vi "Configure Dialog.vi"(2 "First time?":bool) -> ()   [LabVIEW 2016]
uses:
  Communication Global variables.vi
panel:
  in  "REST URL":string="http://10.27.67.2:5800"
  in  "Cancel Button":bool
  in  "Save":bool
  in  "UDP Port":u16=5803
  in  "Robot IP Address":string="10.27.67.2"
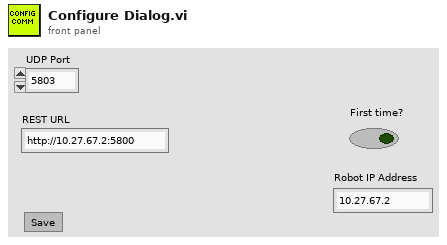
[diagram p1: front panel]
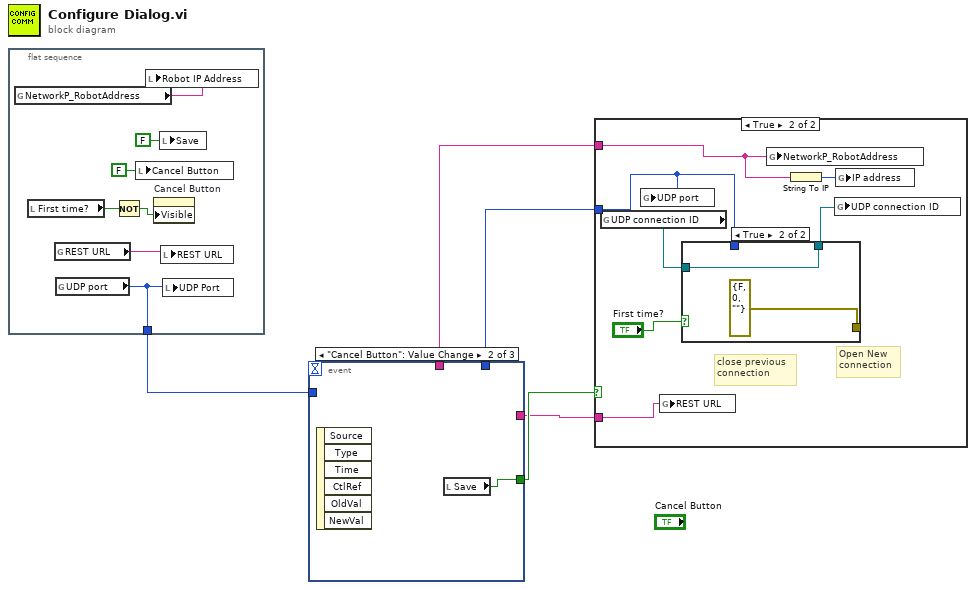
[diagram p0: block diagram]
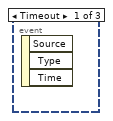
[diagram p2: hidden frame]
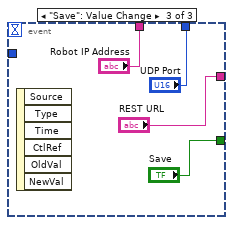
[diagram p3: hidden frame]
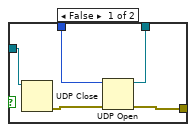
[diagram p5: hidden frame]
diagram:
  n1 = flat-sequence {
    tunnel: [w8] -> w1
    frame #0 {
      n2 = global read "Communication Global variables.vi" "NetworkP_RobotAddress"() -> (w10:string)
      n3 = local read "First time?"() -> (w7:bool)
      n4 = global read "Communication Global variables.vi" "REST URL"() -> (w9:string)
      n5 = global read "Communication Global variables.vi" "UDP port"() -> (w8:u16)
      n6 = Not(x=w7) -> (.not. x?=w6:bool)
      n7 = local write "Cancel Button"(FALSE ("Cancel Button")) -> ()
      n8 = local write "Robot IP Address"(w10) -> ()
      n9 = property on="Cancel Button" class="Bool (strict)"("Visible"=w6) -> ()  [unwired: 2 in, 2 out]
      n10 = local write "Save"(FALSE ("Save")) -> ()
      n11 = local write "REST URL"(w9) -> ()
      n12 = local write "UDP Port"(w8) -> ()
    }
  }
  n13 = event shown="[1] \"Cancel Button\": Value Change" {
    selector: _ -> [_ _ _]
    dyn-events: _ -> [_ _ _]
    timeout: _ -> [_ _ _]
    tunnel: [_ _ "Robot IP Address"] -> w5
    tunnel: [_ _ "UDP Port"] -> w4
    tunnel: [_ w13 "Save"] -> w3
    tunnel: [_ _ "REST URL"] -> w2
    tunnel: w1 -> [_ _ _]
    event Timeout {
      n14 = event-data() -> ()  [unwired: 1 in, 3 out]
    }
    event "Cancel Button": Value Change {
      n15 = event-data() -> ()  [unwired: 1 in, 6 out]
      n16 = local read "Save"() -> (w13:bool)
    }
    event "Save": Value Change {
      n17 = event-data() -> ()  [unwired: 1 in, 6 out]
    }
  }
  n18 = case shown="True" w3 {
    tunnel: w4 -> [_ w19]
    tunnel: w5 -> [_ w18]
    tunnel: w2 -> [_ w22]
    frame False {
    }
    frame True {
      # "Open New \nconnection"
      # "close previous \nconnection"
      n19 = global read "Communication Global variables.vi" "UDP connection ID"() -> (w24:refnum<k16>)
      n20 = global write "Communication Global variables.vi" "UDP port"(w19) -> ()
      n21 = global write "Communication Global variables.vi" "REST URL"(w22) -> ()
      n22 = case shown="True" "First time?" {
        tunnel: w24 -> [w29 w30]
        tunnel: [w28 errorcluster {"status"=FALSE, "code"=0, "source"=""} ("error out")] -> _
        tunnel: [w26 w30] -> w20
        tunnel: w19 -> [w25 _]
        frame False {
          n23 = UDP Close(connection ID=w29) -> (error out=w27:errorcluster)  [unwired: 1 in, 1 out]
          n24 = UDP Open(8:w27, 11:w25) -> (port=w26:refnum<k16>, 0:w28:errorcluster)  [unwired: 3 in, 1 out]
        }
        frame True {
        }
      }
      n25 = global write "Communication Global variables.vi" "NetworkP_RobotAddress"(w18) -> ()
      n26 = String To IP(1:w18) -> (0:w23:u32)
      n27 = global write "Communication Global variables.vi" "UDP connection ID"(w20) -> ()
      n28 = global write "Communication Global variables.vi" "IP address"(w23) -> ()
    }
  }
